vi "ShowItemInProject.vi"(11 "ProjectItem in":refnum<vi>) -> (0 "error out":errorcluster)   [LabVIEW 2020, in "WebView2-Viewer.lvlib"]
uses:
  WebView2-Viewer.lvlib
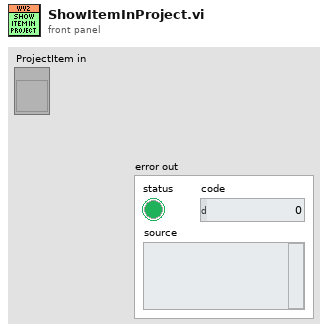
[diagram p1: front panel]
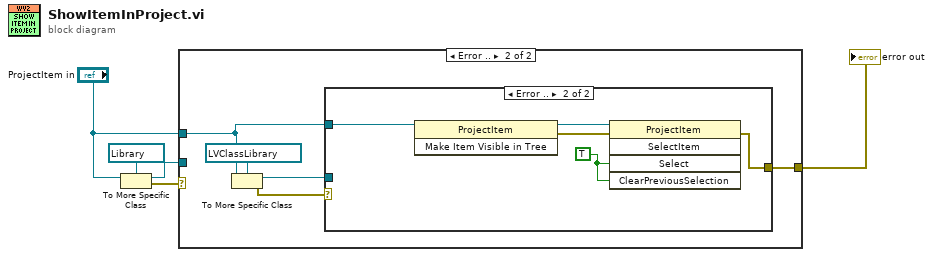
[diagram p0: block diagram]
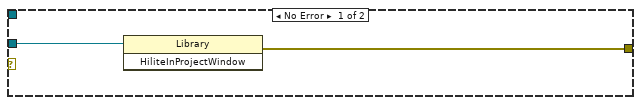
[diagram p2: hidden frame]
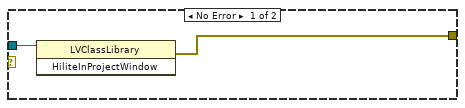
[diagram p3: hidden frame]
diagram:
  n1 = To More Specific Class(target class=refnum<vi> refnum ("reference"), reference="ProjectItem in") -> (specific class reference=w2:refnum<vi>, error out=w3:errorcluster)  [unwired: 1 in]
  n2 = case shown="Error .." w3 {
    tunnel: w2 -> [w7 _]
    tunnel: "ProjectItem in" -> [_ w8]
    tunnel: [w6 w9] -> w5
    frame No Error {
      n3 = invoke class="Library" method="HiliteInProjectWindow"(reference=w7) -> (error out=w6:errorcluster)  [unwired: 2 in, 2 out]
    }
    frame Error {
      n4 = To More Specific Class(target class=refnum<vi> refnum ("reference"), reference=w8) -> (specific class reference=w11:refnum<vi>, error out=w10:errorcluster)  [unwired: 1 in]
      n5 = case shown="Error .." w10 {
        tunnel: w11 -> [w14 _]
        tunnel: [w13 w15] -> w9
        tunnel: w8 -> [_ w16]
        frame No Error {
          n6 = invoke class="LVClassLibrary" method="HiliteInProjectWindow"(reference=w14) -> (error out=w13:errorcluster)  [unwired: 2 in, 2 out]
        }
        frame Error {
          w17 = TRUE ("Select")
          n7 = invoke class="ProjectItem" method="Make Item Visible in Tree"(reference=w16) -> (reference out=w19:refnum<vi>, error out=w18:errorcluster)  [unwired: 2 in, 1 out]
          n8 = invoke class="ProjectItem" method="SelectItem"(reference=w19, error in=w18, "Select"=w17, "ClearPreviousSelection"=w17) -> (error out=w15:errorcluster)  [unwired: 1 in, 4 out]
        }
      }
    }
  }
  "error out" <- w5
